vi "performZeroCalib.vi"(8 "error in (no error)":errorcluster, 10 "command_PerformZeroCalib":T1, 11 "ElectrometerController in":refnum<class "ElectrometerController.lvclass">) -> (0 "error out":errorcluster, 3 "ElectrometerController out":refnum<class "ElectrometerController.lvclass">)   [LabVIEW 2016, in "ElectrometerController.lvclass"]
uses:
  ElectrometerController.lvclass
  ts_sallv_calibrationelectrometer/DataTypes/command_PerformZeroCalib.ctl
  Electrometer/Electrometer.lvclass
  ts_sallv_calibrationelectrometer/SALLV_calibrationElectrometer.lvlib
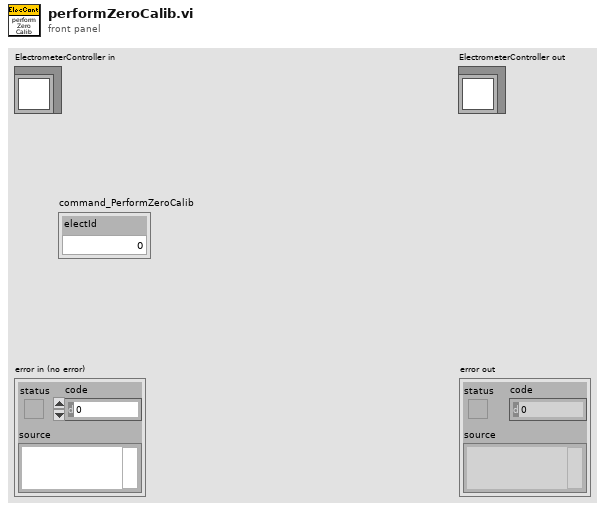
[diagram p1: front panel]
types:
  T1 = typedef "SALLV_calibrationElectrometer.lvlib/command_PerformZeroCalib.ctl" = cluster{"electId":i16}
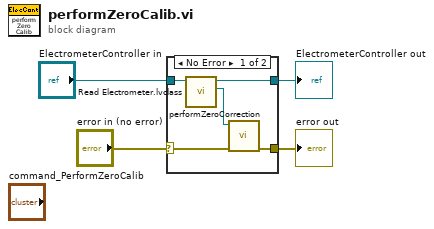
[diagram p0: block diagram]
diagram:
  n1 = case shown="No Error" "error in (no error)" {
    selector: "error in (no error)" -> [w9 w11]
    tunnel: [w8 w11] -> w3
    tunnel: [w5 w10] -> w1
    tunnel: "ElectrometerController in" -> [w7 w10]
    frame No Error {
      n2 = call-dynamic "Read Electrometer.lvclass.vi"("ElectrometerController in"=w7) -> ("Electrometer.lvclass"=w6:refnum<class "Electrometer.lvclass">, "ElectrometerController out"=w5:refnum<class "ElectrometerController.lvclass">)  [unwired: 8 in, 1 out]
      n3 = call "performZeroCorrection.vi"("error in (no error)"=w9, "Electrometer in"=w6) -> ("error out"=w8:errorcluster)  [unwired: 7 in, 2 out]
    }
    frame Error {
    }
  }
  "error out" <- w3
  "ElectrometerController out" <- w1
